vi "getOutputMask.vi"(8 "error in (no error)":errorcluster, 11 "DIO64Output.lvclass in":refnum<class "DIO64Output.lvclass">) -> (0 "error out":errorcluster, 2 "mask":u16[](array[numeric])=[1] format="%.0x", 3 "DIO64Output.lvclass out":refnum<class "DIO64Output.lvclass">)   [LabVIEW 2011, in "Hardware.lvlib" / "Channels.lvlib" / "DIO64Output.lvclass"]
uses:
  DIO64Output.lvclass
  DIO64Output.lvclass/DIO64Output.ctl
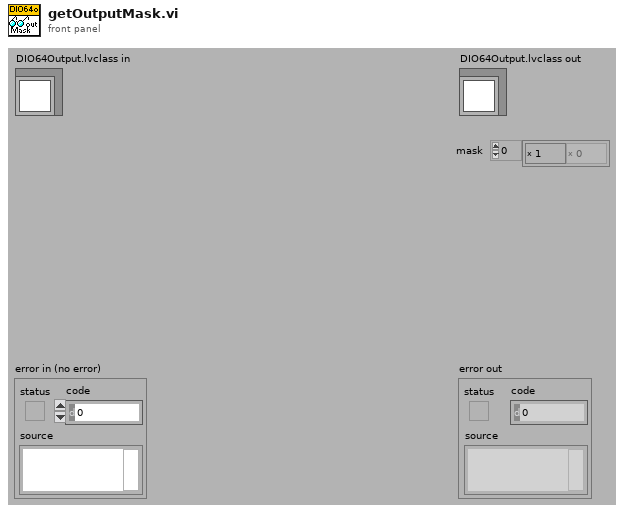
[diagram p1: front panel]
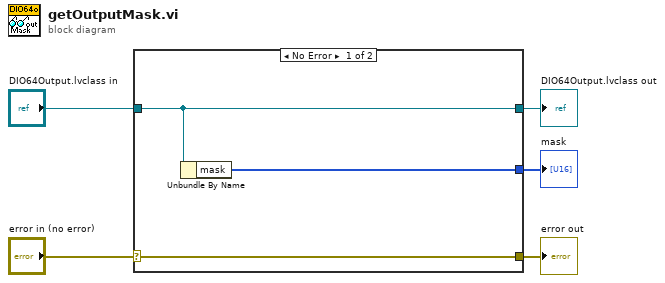
[diagram p0: block diagram]
diagram:
  n1 = case shown="No Error" "error in (no error)" {
    selector: "error in (no error)" -> [w8 w9]
    tunnel: [w8 w9] -> w4
    tunnel: [w7 w10] -> w2
    tunnel: "DIO64Output.lvclass in" -> [w7 w10]
    tunnel: [w6 _] -> w1
    frame No Error {
      n2 = Unbundle By Name(w7) -> ("mask"=w6:u16[])
    }
    frame Error {
    }
  }
  "error out" <- w4
  "DIO64Output.lvclass out" <- w2
  "mask" <- w1
